vi "Read Targets from VIPM Settings.vi"(8 "error in (no error)":errorcluster, 11 "Version Filter":string) -> (0 "error out":errorcluster, 1 "All Targets":T1(array[cluster]), 2 "Port":i32, 3 "Path":path)   [LabVIEW 2019, in "VIPM.lvlib"]
uses:
  VIPM.lvlib
  <vilib>/Utility/sysdir.llb/System Directory Type.ctl
  <vilib>/Utility/config.llb/Read Key (I32).vi
  <vilib>/Utility/config.llb/Read Key (String).vi
  <vilib>/Utility/config.llb/Read Key (Path).vi
  <vilib>/Utility/config.llb/NI_LVConfig.lvlib
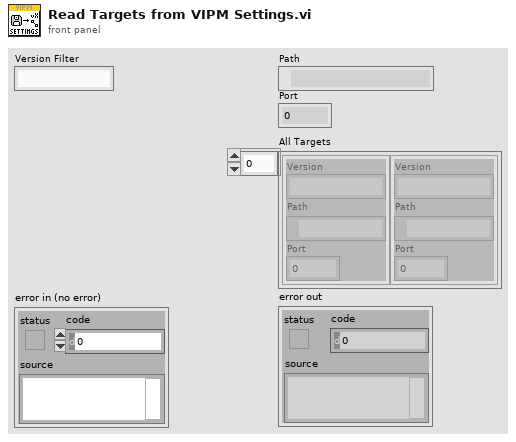
[diagram p1: front panel]
types:
  T1 = cluster{"Version":string, "Path":path, "Port":i32}[]
  T2 = typedef "System Directory Type.ctl" = i32
  T3 = typedef "NI_LVConfig.lvlib/Config Data RefNum.ctl" = refnum<k1>
  T4 = cluster{"Version":string, "Path":path, "Port":i32}
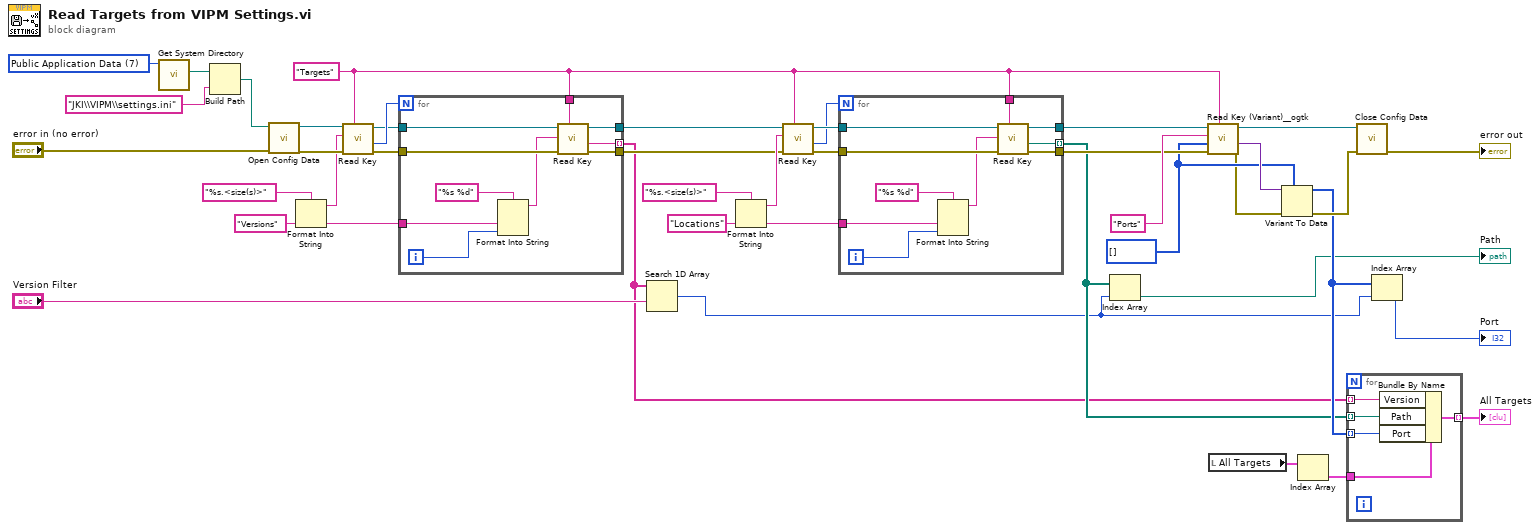
[diagram p0: block diagram]
diagram:
  w12 = i32[] [] ("index of element")
  w23 = "Locations" ("input 1")
  w31 = "Versions" ("input 1")
  w17 = "Targets" ("section")
  w41 = T2 7 items=["User Home"=0, "User Desktop"=1, "User Documents"=2, "User Application Data"=3, "User Preferences"=4, "User Temporary"=5, "Public Documents"=6, "Public Application Data"=7, "Public Preferences"=8, "Public Cache"=13, "System Core Libraries"=9, "System Installed Libraries"=10, "Application Files"=11, "Boot Volume Root"=12] ("system directory type")
  n1 = call <vilib>:"Get System Directory.vi"("system directory type"=w41) -> ("system directory"=w40:path)  [unwired: 10 in]
  n2 = Build Path(base path=w40, name or relative path="JKI\\VIPM\\settings.ini") -> (appended path=w20:path)
  n3 = call <vilib>:"Open Config Data.vi"("error in (no error)"="error in (no error)", "configuration file path"=w20) -> ("error out"=w37:errorcluster, "refnum"=w38:T3)  [unwired: 7 in, 1 out]
  n4 = Format Into String(format string="%s.<size(s)>", w31) -> (resulting string=w35:string)  [unwired: 2 in, 1 out]
  n5 = call-poly <vilib>:"Read Key.vi"("section"=w17, "error in (no error)"=w37, "key"=w35, "refnum"=w38) -> ("error out"=w32:errorcluster, "value"=w34:i32, "refnum out"=w33:T3)  [unwired: 4 in, 1 out]
  n6 = for {
    N: w34 -> [_]
    tunnel: w33 -> [w51]
    tunnel: w32 -> [w50]
    tunnel: w31 -> [w46]
    tunnel: w17 -> [w45]
    tunnel: [w44] -> w26
    tunnel: [w43] -> w25
    tunnel: [w42] -> w4 mode=indexing
    i -> [w47]
    n7 = Format Into String(format string="%s %d", w46, w47) -> (resulting string=w48:string)  [unwired: 2 in, 1 out]
    n8 = call-poly <vilib>:"Read Key.vi"("section"=w45, "error in (no error)"=w50, "key"=w48, "refnum"=w51) -> ("error out"=w43:errorcluster, "value"=w42:string, "refnum out"=w44:T3)  [unwired: 4 in, 1 out]
  }
  n9 = Search 1D Array(1D array=w4, element="Version Filter") -> (index of element=w5:i32)  [unwired: 1 in]
  n10 = Format Into String(format string="%s.<size(s)>", w23) -> (resulting string=w27:string)  [unwired: 2 in, 1 out]
  n11 = call-poly <vilib>:"Read Key.vi"("section"=w17, "error in (no error)"=w25, "key"=w27, "refnum"=w26) -> ("error out"=w30:errorcluster, "value"=w28:i32, "refnum out"=w29:T3)  [unwired: 4 in, 1 out]
  n12 = for {
    N: w28 -> [_]
    tunnel: w29 -> [w61]
    tunnel: w30 -> [w60]
    tunnel: w23 -> [w56]
    tunnel: w17 -> [w55]
    tunnel: [w54] -> w6 mode=indexing
    tunnel: [w53] -> w15
    tunnel: [w52] -> w14
    i -> [w57]
    n13 = Format Into String(format string="%s %d", w56, w57) -> (resulting string=w58:string)  [unwired: 2 in, 1 out]
    n14 = call-poly <vilib>:"Read Key.vi"("section"=w55, "error in (no error)"=w60, "key"=w58, "refnum"=w61) -> ("error out"=w52:errorcluster, "value"=w54:path, "refnum out"=w53:T3)  [unwired: 4 in, 1 out]
  }
  n15 = Index Array(array=w6, index=w5) -> (element=→"Path":path)
  n16 = call <userlib>:"Read Key (Variant)__ogtk.vi"("section"=w17, "error in (no error)"=w14, "type"=w12, "key (optional)"="Ports" ("input 1"), "refnum"=w15) -> ("error out"=w11:errorcluster, "key-value"=w13:variant, "refnum out"=w16:T3)  [unwired: 3 in, 1 out]
  n17 = local read "All Targets"() -> (w9:T1)
  n18 = Variant To Data(error in=w11, type=w12, Variant=w13) -> (data=w7:i32[], error out=w10:errorcluster)
  n19 = Index Array(array=w9) -> (element=w8:T4)  [unwired: 1 in]
  n20 = for {
    tunnel: w8 -> [w66]
    tunnel: w7 -> [w65] mode=indexing
    tunnel: w6 -> [w64] mode=indexing
    tunnel: w4 -> [w63] mode=indexing
    tunnel: [w62] -> w3 mode=indexing
    n21 = Bundle By Name(cluster=w66, "Version"=w63, "Path"=w64, "Port"=w65) -> (w62:T4)
  }
  "All Targets" <- w3
  n22 = call <vilib>:"Close Config Data.vi"("error in (no error)"=w10, "refnum"=w16) -> ("error out"=→"error out":errorcluster)  [unwired: 8 in, 1 out]
  n23 = Index Array(array=w7, index=w5) -> (element=→"Port":i32)
